vi "ExposeSetData.vi"(10 "ExposeDataType":T1, 11 "ExposeID":string) -> ()   [LabVIEW 2017]
uses:
  ExposeDataType.ctl
  ExposeGlobals.vi
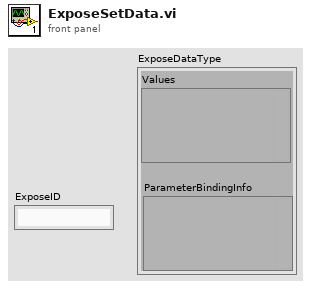
[diagram p1: front panel]
types:
  T1 = typedef "ExposeDataType.ctl" = cluster{"Values":variant, "ParameterBindingInfo":variant}
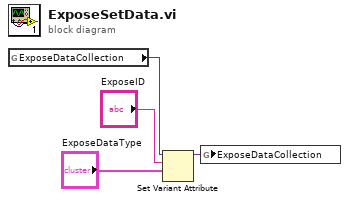
[diagram p0: block diagram]
diagram:
  n1 = global read "ExposeGlobals.vi" "ExposeDataCollection"() -> (w3:variant)
  n2 = Set Variant Attribute(Variant=w3, name="ExposeID", value="ExposeDataType") -> (Variant out=w4:variant)  [unwired: 1 in, 2 out]
  n3 = global write "ExposeGlobals.vi" "ExposeDataCollection"(w4) -> ()
